vi "Resume Timer.vi"(8 "error in (no error)":errorcluster, 11 "Timer in":refnum<class "Timer.lvclass">) -> (0 "error out":errorcluster, 3 "Timer out":refnum<class "Timer.lvclass">)   [LabVIEW 2019, in "Timer.lvlib" / "Timer.lvclass"]
uses:
  Timer.lvclass
  Timer.lvclass/Timer.ctl
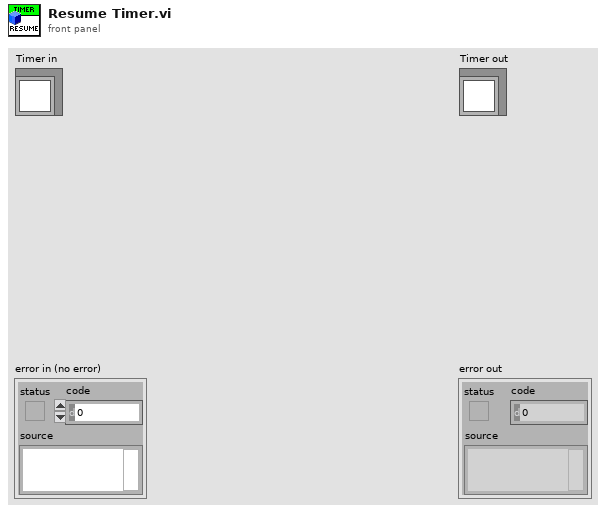
[diagram p1: front panel]
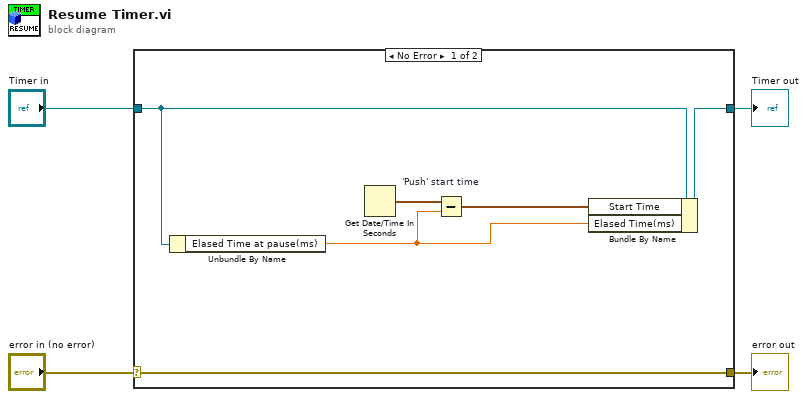
[diagram p0: block diagram]
diagram:
  n1 = case shown="No Error" "error in (no error)" {
    selector: "error in (no error)" -> [w10 w12]
    tunnel: [w10 w12] -> w3
    tunnel: [w7 w11] -> w1
    tunnel: "Timer in" -> [w8 w11]
    frame No Error {
      n2 = Unbundle By Name(w8) -> ("Elased Time at pause(ms)"=w5:dbl)
      n3 = Get Date/Time In Seconds() -> (seconds since 1Jan1904=w9:timestamp)
      n4 = Subtract "'Push' start time"(x=w9, y=w5) -> (x-y=w6:timestamp)
      n5 = Bundle By Name(cluster=w8, "Start Time"=w6, "Elased Time(ms)"=w5) -> (w7:refnum<class "Timer.lvclass">)
    }
    frame Error {
    }
  }
  "error out" <- w3
  "Timer out" <- w1
